vi "Configure Trace Operation (Add,Subtract).vi"(0 "VISA resource name":refnum<visa-resource-name>, 1 "Destination Trace (2: Trace 2)":u16(ring)=2 items=["Trace 1"=1, "Trace 2"=2, "Trace 3"=3], 5 "Trace 1 (1: Trace 1)":u16(ring)=1 items=["Trace 1"=1, "Trace 2"=2, "Trace 3"=3], 7 "Operation (0: Add)":u16(ring) items=["Add", "Subtract"], 9 "Trace 2 (2: Trace 2)":u16(ring)=2 items=["Trace 1"=1, "Trace 2"=2, "Trace 3"=3], 11 "error in (no error)":errorcluster) -> (4 "VISA resource name out":refnum<visa-resource-name>, 15 "error out":errorcluster)   [LabVIEW 2014, in "Agilent ESA PSA Series.lvlib"]
doc: "Adds/Subtracts Trace 1, Trace 2 and Trace 3."
uses:
  Agilent ESA PSA Series.lvlib
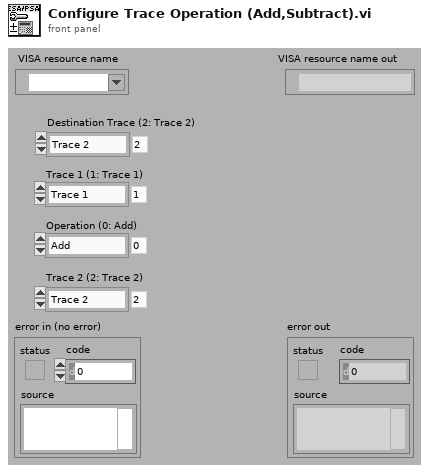
[diagram p1: front panel]
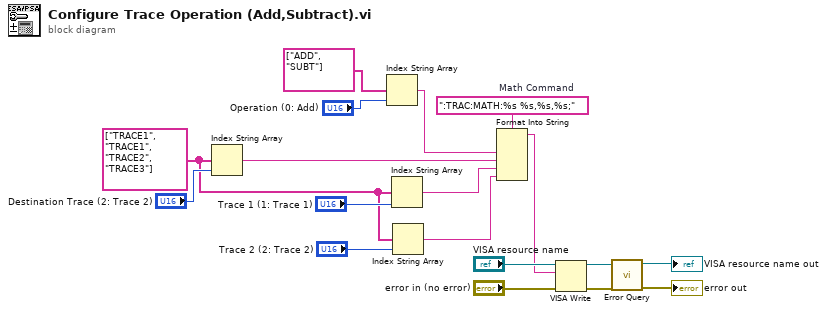
[diagram p0: block diagram]
diagram:
  w9 = ":TRAC:MATH:%s %s,%s,%s;"  # Math Command
  w6 = string[] ["TRACE1", "TRACE1", "TRACE2", "TRACE3"]
  n1 = Index String Array(1:"Destination Trace (2: Trace 2)", 2:w6) -> (0:w5:string)  [unwired: 1 in]
  n2 = Index String Array(1:"Operation (0: Add)", 2:string[] ["ADD", "SUBT"]) -> (0:w4:string)  [unwired: 1 in]
  n3 = Index String Array(1:"Trace 1 (1: Trace 1)", 2:w6) -> (0:w3:string)  [unwired: 1 in]
  n4 = Index String Array(1:"Trace 2 (2: Trace 2)", 2:w6) -> (0:w2:string)  [unwired: 1 in]
  n5 = Format Into String(format string=w9, w4, w5, w3, w2) -> (resulting string=w1:string)  [unwired: 2 in, 1 out]
  n6 = VISA Write(VISA resource name="VISA resource name", write buffer=w1, error in (no error)="error in (no error)") -> (VISA resource name out=w16:refnum<visa-resource-name>, error out=w14:errorcluster)  [unwired: 1 out]
  n7 = call "Error Query.vi"("error in (no error)"=w14, "VISA resource name"=w16) -> ("error out"=→"error out":errorcluster, "VISA resource name out"=→"VISA resource name out":refnum<visa-resource-name>)  [unwired: 6 in, 2 out]
